vi "Configure Trigger (Ethernet - QTAG).vi"(0 "VISA resource name":refnum<visa-resource-name>, 5 "Trigger Source (9: Bus 1)":u16(ring)=9 items=["Bus 1"=9, "Bus 2"=10], 7 "QTAG Value (\"XXXXXXXX\")":string="XXXXXXXX", 11 "error in (no error)":errorcluster) -> (4 "VISA resource name out":refnum<visa-resource-name>, 15 "error out":errorcluster)   [LabVIEW 2009, in "Tektronix DPO MSO 2000 4000 Series.lvlib"]
doc: "Configures QTAG trigger settings for Ethernet trigger. \n\n<B>Note:</B>\nThis VI only applies to DPO4034B, DPO4054B, DPO4104B, MSO4034B, MSO4054B, MSO4104B."
uses:
  <instrlib>/Tektronix DPO MSO 2000 4000 Series/Tektronix DPO MSO 2000 4000 Series.lvlib
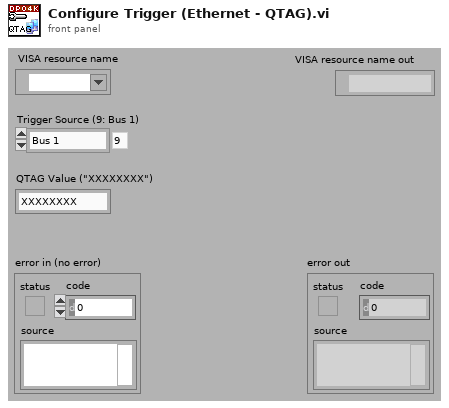
[diagram p1: front panel]
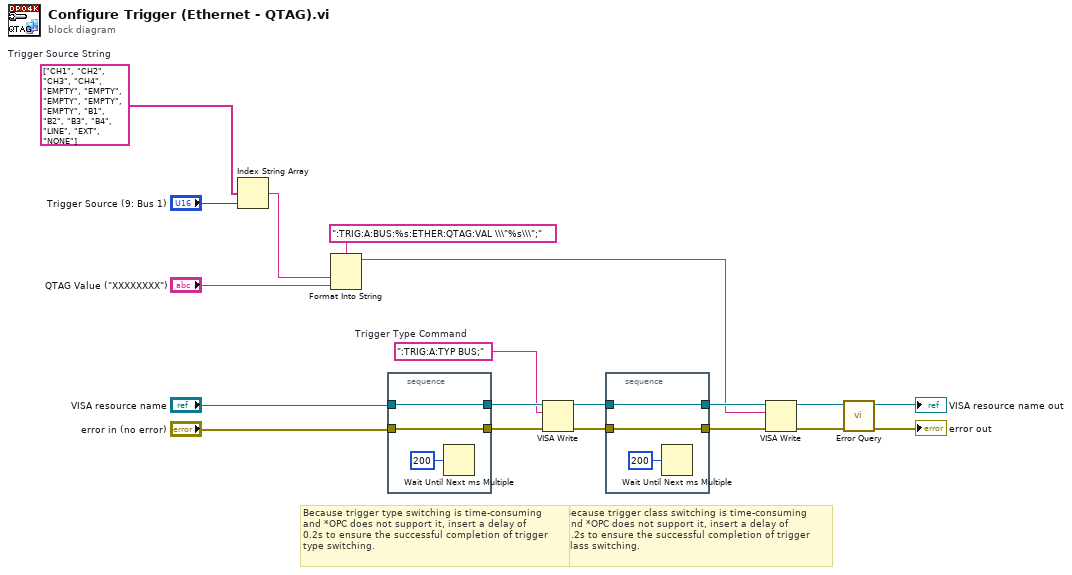
[diagram p0: block diagram]
diagram:
  w12 = string[] ["CH1", "CH2", "CH3", "CH4", "EMPTY", "EMPTY", "EMPTY", "EMPTY", "EMPTY", "B1", "B2", "B3", "B4", "LINE", "EXT", "NONE"]  # Trigger Source String
  w17 = ":TRIG:A:TYP BUS;"  # Trigger Type Command
  # "Because trigger class switching is time-consuming\nand *OPC does not support it, insert a delay of\n0.2s to ensure the successful completion of trigger\nclass switching."
  # "Because trigger type switching is time-consuming\nand *OPC does not support it, insert a delay of\n0.2s to ensure the successful completion of trigger\ntype switching."
  n1 = Index String Array(1:"Trigger Source (9: Bus 1)", 2:w12) -> (0:w2:string)  [unwired: 1 in]
  n2 = Format Into String(format string=":TRIG:A:BUS:%s:ETHER:QTAG:VAL \\\"%s\\\";", w2, "QTAG Value (\"XXXXXXXX\")") -> (resulting string=w1:string)  [unwired: 2 in, 1 out]
  n3 = stacked-sequence {
    tunnel: "VISA resource name" -> [w21]
    tunnel: [w21] -> w19
    tunnel: "error in (no error)" -> [w20]
    tunnel: [w20] -> w18
    frame #0 {
      n4 = Wait Until Next ms Multiple(millisecond multiple=u32 200) -> ()  [unwired: 1 out]
    }
  }
  n5 = VISA Write(VISA resource name=w19, write buffer=w17, error in (no error)=w18) -> (VISA resource name out=w16:refnum<visa-resource-name>, error out=w15:errorcluster)  [unwired: 1 out]
  n6 = stacked-sequence {
    tunnel: w16 -> [w24]
    tunnel: [w24] -> w14
    tunnel: w15 -> [w23]
    tunnel: [w23] -> w13
    frame #0 {
      n7 = Wait Until Next ms Multiple(millisecond multiple=u32 200) -> ()  [unwired: 1 out]
    }
  }
  n8 = VISA Write(VISA resource name=w14, write buffer=w1, error in (no error)=w13) -> (VISA resource name out=w10:refnum<visa-resource-name>, error out=w9:errorcluster)  [unwired: 1 out]
  n9 = call <instrlib>:"Error Query.vi"("error in (no error)"=w9, "VISA resource name"=w10) -> ("error out"=→"error out":errorcluster, "VISA resource name out"=→"VISA resource name out":refnum<visa-resource-name>)  [unwired: 6 in, 2 out]
